vi "get cal data.vi"(8 "error in (no error)":errorcluster, 10 "cal file path":path, 11 "device_type in":refnum<class "device_type.lvclass">) -> (0 "error out":errorcluster, 3 "device_type out":refnum<class "device_type.lvclass">)   [LabVIEW 2021, in "device_type.lvclass"]
uses:
  device_type.lvclass
  device_type.lvclass/device_type.ctl
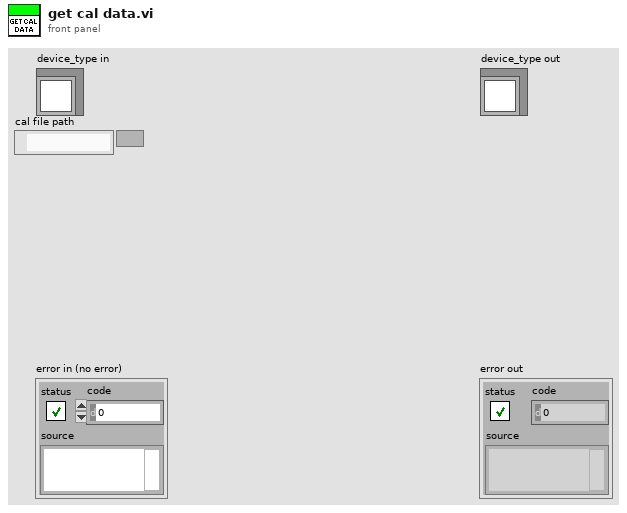
[diagram p1: front panel]
types:
  T1 = enum16{"open", "open or create", "create or replace", "create", "open (read-only)"}
  T2 = cluster{"freqency":dbl[], "phase":dbl[], "amp":dbl[]}
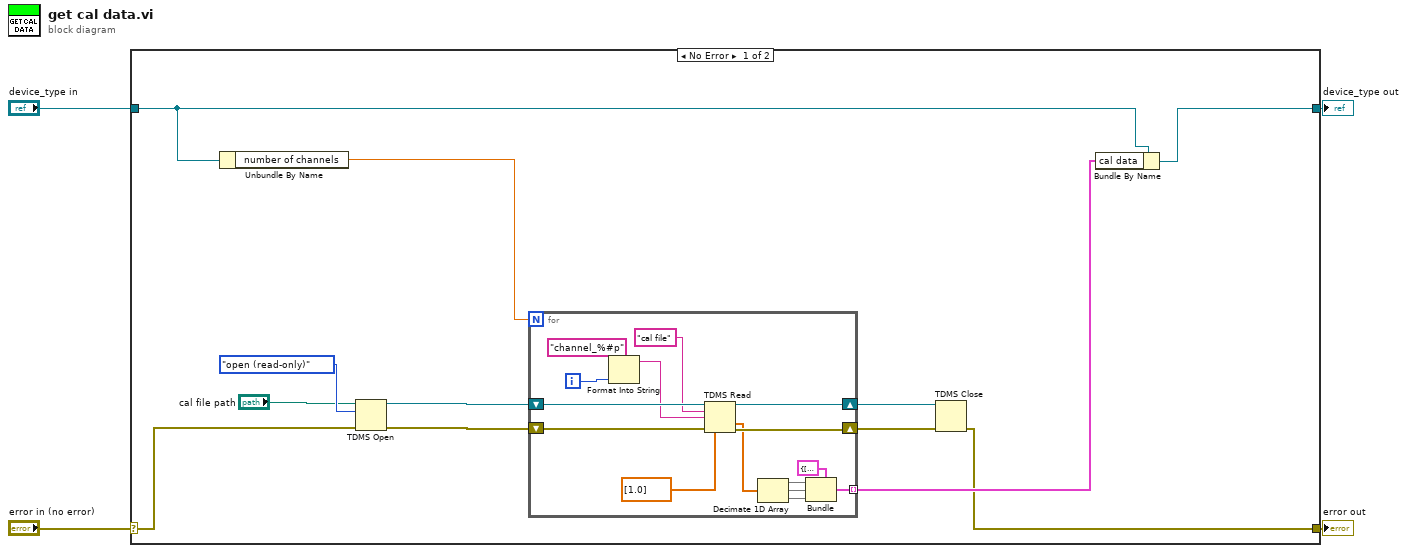
[diagram p0: block diagram]
diagram:
  n1 = case shown="No Error" "error in (no error)" {
    selector: "error in (no error)" -> [w6 w33]
    tunnel: [w5 w33] -> w3
    tunnel: [w8 w32] -> w1
    tunnel: "device_type in" -> [w9 w32]
    frame No Error {
      n2 = Unbundle By Name(w9) -> ("number of channels"=w10:dbl)
      n3 = TDMS Open(8:w6, 10:T1."open (read-only)" ("operation (0:open)"), 11:"cal file path") -> (0:w15:errorcluster, 3:w16:refnum<k34>)  [unwired: 4 in]
      n4 = for {
        N: w10 -> [_]
        shift-right: [w29] -> w14
        shift-left: w16 -> [w31]
        shift-right: [w28] -> w13
        shift-left: w15 -> [w30]
        tunnel: [w17] -> w7 mode=indexing
        i -> [w27]
        n5 = Format Into String(format string="channel_%#p", w27) -> (resulting string=w25:string)  [unwired: 2 in, 1 out]
        n6 = TDMS Read(0:w31, 5:"cal file" ("group name in (Untitled)"), 7:w25, 11:w30, 12:dbl[] [1.0] ("interleaved array")) -> (4:w29:refnum<k34>, 10:w22:dbl[], 15:w28:errorcluster)  [unwired: 3 in, 3 out]
        n7 = Decimate 1D Array(w22) -> (w20:dbl[], w19:dbl[], w18:dbl[])
        n8 = Bundle(cluster=T2 {"freqency"=[], "phase"=[], "amp"=[]}, "freqency"=w20, "phase"=w19, "amp"=w18) -> (w17:T2)
      }
      n9 = TDMS Close(8:w13, 11:w14) -> (0:w5:errorcluster)  [unwired: 1 out]
      n10 = Bundle By Name(cluster=w9, "cal data"=w7) -> (w8:refnum<class "device_type.lvclass">)
    }
    frame Error {
    }
  }
  "error out" <- w3
  "device_type out" <- w1
